vi "CheckNumberOfPhases.vi"(8 "error in (no error)":errorcluster, 11 "NHRGridSim in":refnum<class "NHRGridSim.lvclass">) -> (0 "error out":errorcluster, 1 "NumberOfPhases":i32, 2 "Boolean":bool, 3 "NHRGridSim out":refnum<class "NHRGridSim.lvclass">)   [LabVIEW 2018, in "AcPwrPlugins.lvlib" / "NHRGridSim.lvclass"]
doc: "This VI checks the number of phases and ensures that it is less than or equal to three."
uses:
  NHRGridSim.lvclass
  <vilib>/Utility/error.llb/Error Cluster From Error Code.vi
  <vilib>/ErrorRing/Error Ring.xnode
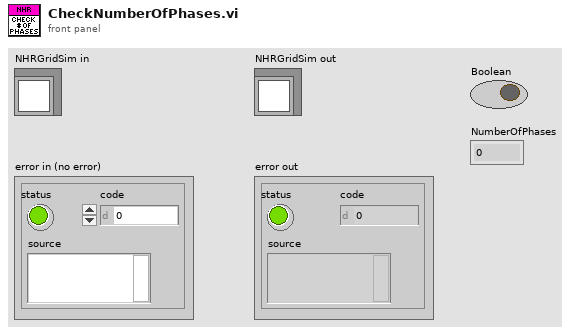
[diagram p1: front panel]
types:
  T1 = typedef "AcPwrPlugins.lvlib/NHRGridSim.lvclass/Modules.ctl" = cluster{"Measurement":cluster{"ApertureLength (s)":dbl, "NumberOfSamples":u32}, "Ranges":cluster{"Irange (A)":dbl, "Vrange (V)":dbl}, "Mode":u8, "Handle":string, "FreqOut (Hz)":dbl, "Connected":bool, "btnIdQuery":bool, "btnReset":bool, "Initialize Timeout ( ms)":u32, "Phase (0: All)":i32, "WatchDog":cluster{"Enable WatchDog":bool, "Robust WatchDog":bool, "Watchdog Interval (s)":dbl}, "Safety Limits":cluster{"Min Voltage (V)":dbl, "Min Voltage Time (s)":dbl, "Max Voltage (V)":dbl, "MaxVoltage Time (s)":dbl, "Max Source Amps (A)":dbl, "Max Source Amps Time (s)":dbl, "Max Sink Amps (A)":dbl, "Max Sink Amps Time (s)":dbl, "Max Source Power (W)":dbl, "Max Source Power Time (s)":dbl, "Max Sink Power (W)":dbl, "Max Sink Power Time (s)":dbl, "Peak Voltage (V)":dbl, "Peak Voltage Enable":bool, "Peak Amps (A)":dbl, "Peak Amps Enable":bool}, "Phases":cluster{"Pout (W)":dbl, "Iout (A)":dbl, "PhaseAngle":dbl, "Vout (V)":dbl, "Phase Name":string}[], "Regulation Gain":dbl, "ChangeOntheFly":bool, "Synchronize Output \nto Phase":bool, "Slew Rate":cluster{"Voltage Slew (Volts/s)":dbl, "Phase Angle (Degrees/s)":dbl}}[]
  T2 = cluster{"Pout (W)":dbl, "Iout (A)":dbl, "PhaseAngle":dbl, "Vout (V)":dbl, "Phase Name":string}[]
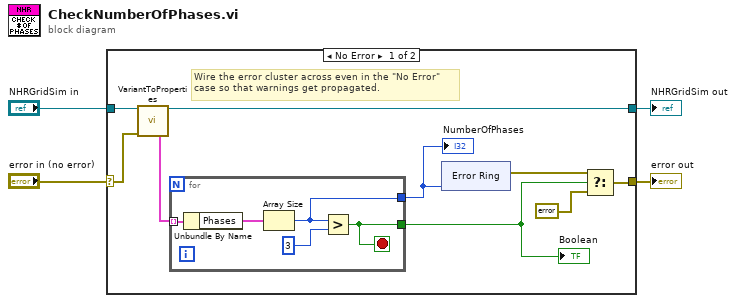
[diagram p0: block diagram]
diagram:
  n1 = case shown="No Error" "error in (no error)" {
    selector: "error in (no error)" -> [w6 w27]
    tunnel: [w9 w27] -> w3
    tunnel: [w7 w26] -> w1
    tunnel: "NHRGridSim in" -> [w8 w26]
    frame No Error {
      # "Wire the error cluster across even in the \"No Error\"\ncase so that warnings get propagated."
      n2 = call "VariantToProperties.vi"("NHRGridSim in"=w8, "error in (no error)"=w6) -> ("NHRGridSim out"=w7:refnum<class "NHRGridSim.lvclass">, "Modules"=w5:T1)  [unwired: 7 in, 5 out]
      n3 = for {
        tunnel: w5 -> [w23] mode=indexing
        tunnel: [w22] -> w10
        tunnel: [w21] -> w13
        stop <- w22 stop-if-true
        n4 = Unbundle By Name(w23) -> ("Phases"=w25:T2)
        n5 = Array Size(array=w25) -> (size(s)=w21:i32)
        n6 = Greater?(x=w21, y=3) -> (0:w22:bool)
      }
      "NumberOfPhases" <- w13
      "Boolean" <- w10
      n7 = xnode "Error Ring"("parameter 0"=w13) -> ("error out"=w12:errorcluster)
      n8 = Select(t=w12, s=w10, f=errorcluster {"status"=FALSE, "code"=0, "source"=""}) -> (s? t:f=w9:errorcluster)
    }
    frame Error {
    }
  }
  "error out" <- w3
  "NHRGridSim out" <- w1
